vi "FTW-Connector-Connect.vi"(0 "FTW Actor Connector Type":refnum<class "FTW-ActorConnector.lvclass">, 5 "Instance Inbox Address":T1, 11 "error in":errorcluster) -> (4 "FTW Actor Connector":refnum<class "FTW-ActorConnector.lvclass">, 15 "error out":errorcluster)   [LabVIEW 2012, in "FTW-Actor.lvlib" / "FTW-ActorConnector.lvclass"]
uses:
  FTW-ActorConnector.lvclass
  Utility/FTW-Actor-Address.ctl
  FTW-ActorConnector.lvclass/FTW-ActorConnector.ctl
  Ether/FTW-Ether.lvclass
  FTW-Actor.lvlib
panel:
  # "Inputs"
  # "Outputs"
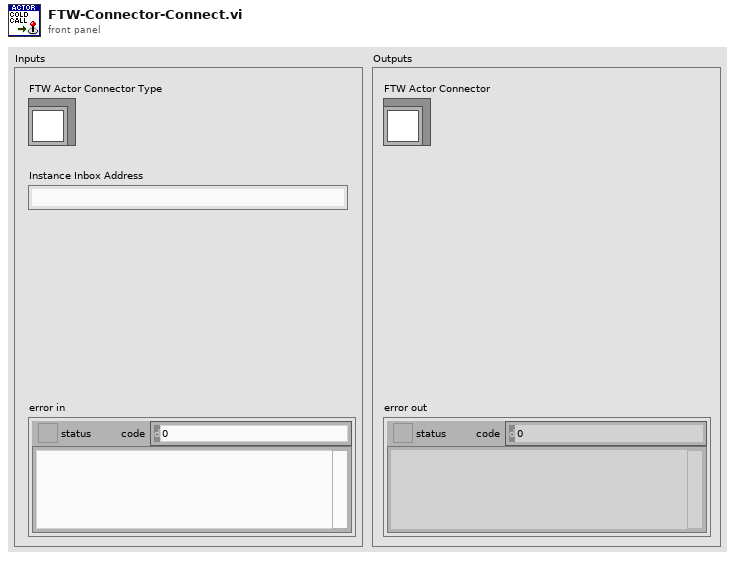
[diagram p1: front panel]
types:
  T1 = typedef "FTW-Actor.lvlib/FTW-Actor-Address.ctl" = string
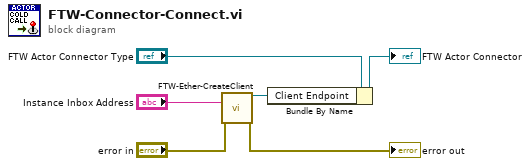
[diagram p0: block diagram]
diagram:
  n1 = call "FTW-Ether-CreateClient.vi"("Server Address"="Instance Inbox Address", "error in"="error in") -> ("Client Endpoint"=w1:refnum<class "FTW-Endpoint.lvclass">, "error out"=→"error out":errorcluster)  [unwired: 12 in]
  n2 = Bundle By Name(cluster="FTW Actor Connector Type", "Client Endpoint"=w1) -> (→"FTW Actor Connector":refnum<class "FTW-ActorConnector.lvclass">)
